vi "Power Output Build Key Array for Config.vi"(8 "error in (no error)":errorcluster, 9 "Power Output Test Parameters":T2={"Stimulus"={"Frequency Type"=enum."Band Edges", "Frequency Ranges"=[], "TX 1 Frequency (MHz)"={"Min"=0.0, "Max"=0.0}, "TX 2 Frequency (MHz)"={"Min"=0.0, "Max"=0.0}, "RX Frequency (MHz)"={"Min"=0.0, "Max"=0.0}, "Pad Model Number"="", "Pad Serial Number"="", "Pad Values"=[]}, "Measurement"={"DUT Port"=enum."Port 1", "Direction"=0, "Frequency Step Size"=0}, "Display"={"Frequency"={"Min"=-1.0, "Max"=-1.0}, "Power"={"Min"=-1, "Max"=-1}}, "Limit"={"Min Power (dBm)"=44.0}, "Calibration"={"Calibrated?"=FALSE}} {"Measurement"."Frequency Step Size" items=["0.2", "0.4", "1.0", "2.0", "4.0"]; "Measurement"."Direction" items=["Reverse", "Forward", "Auxiliary"]}, 10 "Key Array In":T11, 11 "Connection Refnum":T1) -> (0 "error out":errorcluster, 2 "Key Array Out":T11, 3 "Connection Refnum":T1)   [LabVIEW 2011]
uses:
  ITK EXT/utils/keyedarr.llb/Keyed Array.ctl
  TypeDefs/Power Output Test Parameters.ctl
  TypeDefs/Power Output Stimulus Parameters.ctl
  TypeDefs/Power Output Measurement Parameters.ctl
  BPIMCore EXT/HW IO/DUTport.ctl
  BPIMCore EXT/HW IO/MeasMode.ctl
  BPIMCore EXT/HW IO/PIM Sweep Step Size.ctl
  TypeDefs/Power Output Display Parameters.ctl
  TypeDefs/Power Output Limit Parameters.ctl
  TypeDefs/Power Output Calibration State.ctl
  Summitek EXT/ODBC/SQL Controls/Connection Refnum.ctl
  ITK EXT/utils/strutil.llb/Case Matching.ctl
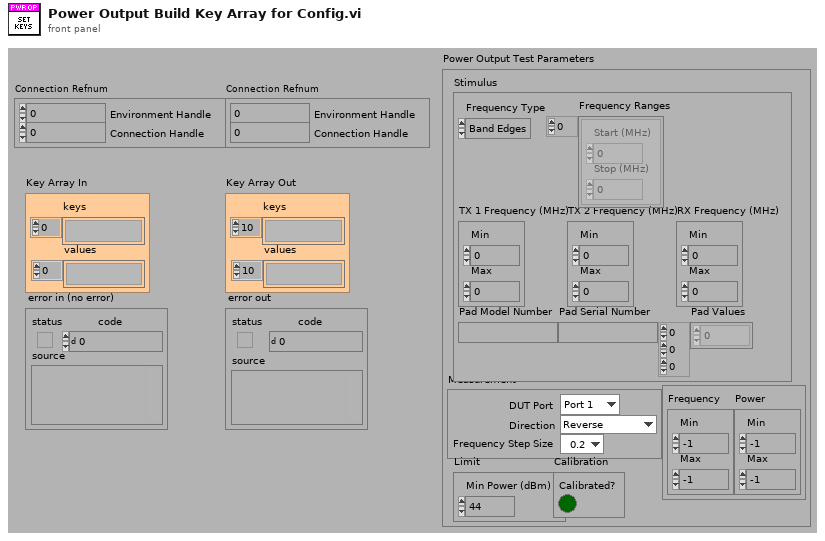
[diagram p1: front panel]
types:
  T1 = typedef "Connection Refnum.ctl" = cluster{"Environment Handle":i32, "Connection Handle":i32}
  T2 = typedef "Power Output Test Parameters.ctl" = cluster{"Stimulus":T3, "Measurement":T4, "Display":T8, "Limit":T9, "Calibration":T10}
  T3 = typedef "Power Output Stimulus Parameters.ctl" = cluster{"Frequency Type":enum16{"Band Edges", "Custom"}, "Frequency Ranges":cluster{"Start (MHz)":dbl, "Stop (MHz)":dbl}[], "TX 1 Frequency (MHz)":cluster{"Min":dbl, "Max":dbl}, "TX 2 Frequency (MHz)":cluster{"Min":dbl, "Max":dbl}, "RX Frequency (MHz)":cluster{"Min":dbl, "Max":dbl}, "Pad Model Number":string, "Pad Serial Number":string, "Pad Values":dbl[][][]}
  T4 = typedef "Power Output Measurement Parameters.ctl" = cluster{"DUT Port":T5, "Direction":T6, "Frequency Step Size":T7}
  T5 = typedef "DUTport.ctl" = enum16{"Port 1", "Port 2"}
  T6 = typedef "MeasMode.ctl" = u16
  T7 = typedef "PIM Sweep Step Size.ctl" = u16
  T8 = typedef "Power Output Display Parameters.ctl" = cluster{"Frequency":cluster{"Min":dbl, "Max":dbl}, "Power":cluster{"Min":i32, "Max":i32}}
  T9 = typedef "Power Output Limit Parameters.ctl" = cluster{"Min Power (dBm)":dbl}
  T10 = typedef "Power Output Calibration State.ctl" = cluster{"Calibrated?":bool}
  T11 = typedef "Keyed Array.ctl" = cluster{"keys":string[], "values":string[]}
  T12 = typedef "Case Matching.ctl" = enum16{"a != A", "a == A", "system"}
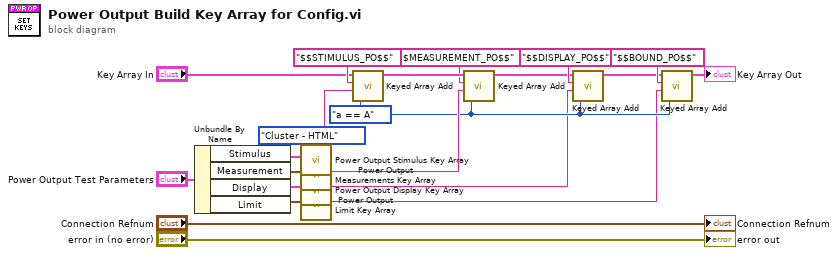
[diagram p0: block diagram]
diagram:
  w11 = Case_Matching."a == A" ("case matching (sensitive)")
  w10 = enum16{"Cluster - HTML", "HTML - Cluster"}."Cluster - HTML" ("Conversion")
  n1 = Unbundle By Name("Power Output Test Parameters") -> ("Stimulus"=w13:T3, "Measurement"=w12:T4, "Display"=w1:T8, "Limit"=w2:T9)
  n2 = call "Power Output Stimulus Key Array.vi"("Conversion"=w10, "Stimulus Cluster In"=w13) -> ("Stimulus HTML Out"=w18:string)  [unwired: 5 in, 1 out]
  n3 = call "Power Output Measurements Key Array.vi"("Conversion"=w10, "Measurements Cluster In"=w12) -> ("Measurements HTML Out"=w16:string)  [unwired: 5 in, 1 out]
  n4 = call "Power Output Display Key Array.vi"("Conversion"=w10, "Display Cluster In"=w1) -> ("Display HTML Out"=w4:string)  [unwired: 5 in, 1 out]
  n5 = call "Power Output Limit Key Array.vi"("Conversion"=w10, "Limits Cluster In"=w2) -> ("Limits HTML Out"=w3:string)  [unwired: 5 in, 1 out]
  n6 = call "Keyed Array Add.vi"("case matching (sensitive)"=w11, "value"=w18, "key"="$$STIMULUS_PO$$", "array in"="Key Array In") -> ("array out"=w20:T11)  [unwired: 3 out]
  n7 = call "Keyed Array Add.vi"("case matching (sensitive)"=w11, "value"=w16, "key"="$$MEASUREMENT_PO$$", "array in"=w20) -> ("array out"=w5:T11)  [unwired: 3 out]
  n8 = call "Keyed Array Add.vi"("case matching (sensitive)"=w11, "value"=w4, "key"="$$DISPLAY_PO$$", "array in"=w5) -> ("array out"=w6:T11)  [unwired: 3 out]
  n9 = call "Keyed Array Add.vi"("case matching (sensitive)"=w11, "value"=w3, "key"="$$BOUND_PO$$", "array in"=w6) -> ("array out"=→"Key Array Out":T11)  [unwired: 3 out]
  "error out" <- "error in (no error)"
  "Connection Refnum" <- "Connection Refnum"
